vi "WSS_Data_Conversion.vi"(9 "WD":sgl, 10 "PPR":sgl, 11 "Speed":sgl) -> (2 "Inactive":u32, 3 "Active":u32)   [LabVIEW 2017, in "FPGA Addon Engine.lvlib"]
uses:
  FPGA Addon Engine.lvlib
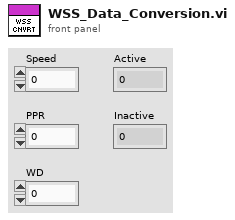
[diagram p1: front panel]
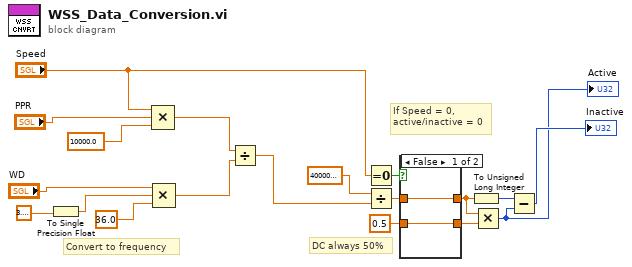
[diagram p0: block diagram]
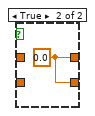
[diagram p2: hidden frame]
diagram:
  # "Convert to frequency"
  # "If Speed = 0, \nactive/inactive = 0"
  # "DC always 50%"
  n1 = To Single Precision Float(number=3.141592653589793) -> (single precision float=w5:sgl)
  n2 = Compound Arithmetic op=MULTIPLY("Speed", "PPR", sgl 10000.0 ("value")) -> (w3:sgl)
  n3 = Compound Arithmetic op=MULTIPLY("WD", w5, sgl 36.0 ("value")) -> (w2:sgl)
  n4 = Divide(x=w3, y=w2) -> (x/y=w1:sgl)
  n5 = Equal To 0?(x="Speed") -> (x = 0?=w15:bool)
  n6 = Divide(x=sgl 40000000.0 ("y"), y=w1) -> (x/y=w17:sgl)
  n7 = case shown="False" w15 {
    tunnel: [w21 w22] -> w16
    tunnel: w17 -> [w21 _]
    tunnel: [w20 w22] -> w18
    tunnel: sgl 0.5 -> [w20 _]
    frame False {
    }
    frame True {
      w22 = sgl 0.0
    }
  }
  n8 = To Unsigned Long Integer(number=w16) -> (unsigned 32bit integer=w11:u32)
  n9 = Multiply(x=w16, y=w18) -> (x*y=w13:u32)
  "Active" <- w13
  n10 = Subtract(x=w11, y=w13) -> (x-y=→"Inactive":u32)
